vi "SSC DCPower Configure Power Line Frequency.vi"(0 "DCPower SSC in":T2[](array[typedef]), 5 "Power Line Frequency":T1=60.0 items=["50 Hertz"=50.0, "60 Hertz"=60.0], 11 "error in":errorcluster) -> (4 "DCPower SSC out":T2[](array[typedef]), 15 "error out":errorcluster)   [LabVIEW 2020]
doc: "This VI configures the power line frequency of the sessions."
uses:
  SSC DCPower.ctl
  <instrlib>/niDCPower/nidcpower.llb/niDCPower Power Line Frequency.ctl
  SSC DCPower Debug Global.vi
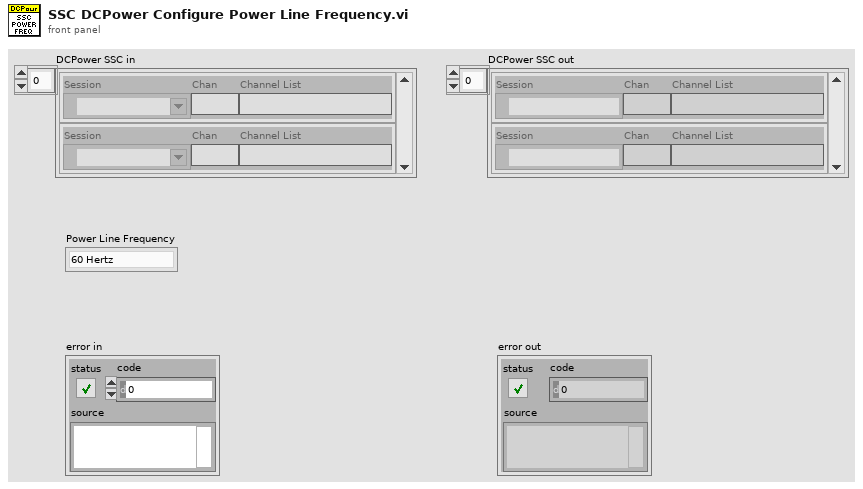
[diagram p1: front panel]
types:
  T1 = typedef "niDCPower Power Line Frequency.ctl" = dbl
  T2 = typedef "SSC DCPower.ctl" = cluster{"Session":refnum<k15>, "Chan":string, "Channel List":string}
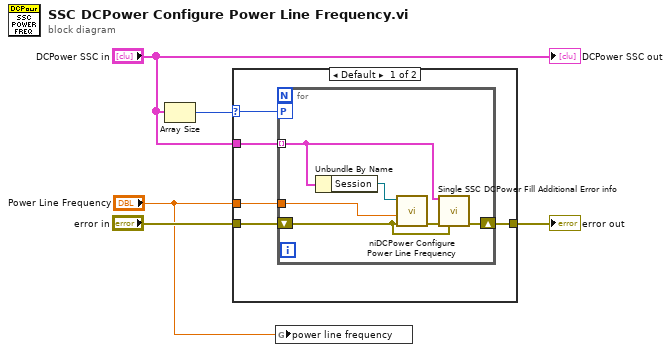
[diagram p0: block diagram]
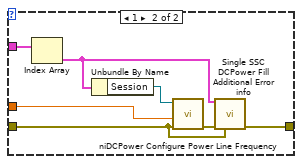
[diagram p2: hidden frame]
diagram:
  n1 = Array Size(array="DCPower SSC in") -> (size(s)=w3:i32)
  n2 = case shown="Default" w3 {
    selector: w3 -> [w8 _]
    tunnel: [w10 w23] -> w5
    tunnel: "error in" -> [w9 w17]
    tunnel: "DCPower SSC in" -> [w7 w22]
    tunnel: "Power Line Frequency" -> [w6 w21]
    frame Default {
      n3 = for {
        tunnel: w7 -> [w12] mode=indexing
        workers-P: w8 -> [_]
        tunnel: w6 -> [w16]
        shift-right: [w13] -> w10
        shift-left: w9 -> [w11]
        n4 = Unbundle By Name(w12) -> ("Session"=w14:refnum<k15>)
        n5 = call <instrlib>:"niDCPower Configure Power Line Frequency.vi"("error in (no error)"=w11, "power line frequency"=w16, "instrument handle"=w14) -> ("error out"=w15:errorcluster)  [unwired: 7 in, 1 out]
        n6 = call "Single SSC DCPower Fill Additional Error info.vi"("DCPower SSC in"=w12, "error in"=w15, "previous error in"=w11) -> ("error out"=w13:errorcluster)  [unwired: 12 in]
      }
    }
    frame 1 {
      n7 = Index Array(array=w22) -> (element=w18:T2)  [unwired: 1 in]
      n8 = Unbundle By Name(w18) -> ("Session"=w19:refnum<k15>)
      n9 = call <instrlib>:"niDCPower Configure Power Line Frequency.vi"("error in (no error)"=w17, "power line frequency"=w21, "instrument handle"=w19) -> ("error out"=w20:errorcluster)  [unwired: 7 in, 1 out]
      n10 = call "Single SSC DCPower Fill Additional Error info.vi"("DCPower SSC in"=w18, "error in"=w20, "previous error in"=w17) -> ("error out"=w23:errorcluster)  [unwired: 12 in]
    }
  }
  "error out" <- w5
  n11 = global write "SSC DCPower Debug Global.vi" "power line frequency"("Power Line Frequency") -> ()
  "DCPower SSC out" <- "DCPower SSC in"
